vi "I16_Type To Enum.vi"(11 "Default":i16) -> (3 "Data Type Enum":T1)   [LabVIEW 2020, in "Current Value Table(Rebuild).lvlib"]
doc: "This VI takes a data type and returns the enum value associated with this data type. This is used during the save process to regenerate the tag listing."
uses:
  Current Value Table(Rebuild).lvlib
  Type Defs/Data Types.ctl
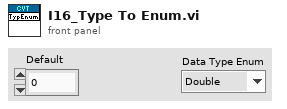
[diagram p1: front panel]
types:
  T1 = typedef "Current Value Table(Rebuild).lvlib/Data Types.ctl" = enum16{"Double", "Single", "I64", "I32", "I16", "I8", "U64", "U32", "U16", "U8", "String", "Boolean", "Array of U8", "Array of U16", "Array of U32", "Array of U64", "Array of I64", "Array of I32", "Array of I16", "Array of I8", "Array of Double", "Array of Single", "Array of Boolean", "Array of String"}
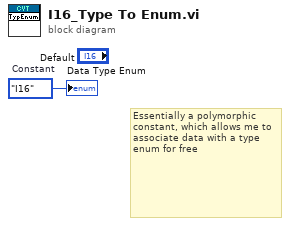
[diagram p0: block diagram]
diagram:
  w1 = Data_Types."I16"  # Constant
  # "Essentially a polymorphic constant, which allows me to associate data with a type enum for free"
  "Data Type Enum" <- w1
